vi "Argmin_min.vi"(6 "Type Y":enum16{"Array", "Sparse"}(ring), 7 "Type X":enum16{"Array", "Sparse"}(ring), 8 "error in":errorcluster caption="entrée d'erreur", 9 "Y":string[][](array[string]), 10 "X":string[][](array[string]), 11 "pairwise_distances_argmin_min":T2={"axis"=1, "metric "="euclidean", "metric_kwargs"={"metric"=[], "kwargs"=[]}, "Returns"="argmin"}) -> (0 "error out":errorcluster caption="sortie d'erreur", 3 "Data":T1)   [LabVIEW 2020]
uses:
  Argmin_min.lvclass
panel:
  out "Argmin_min.lvclass":refnum<class "Argmin_min.lvclass">
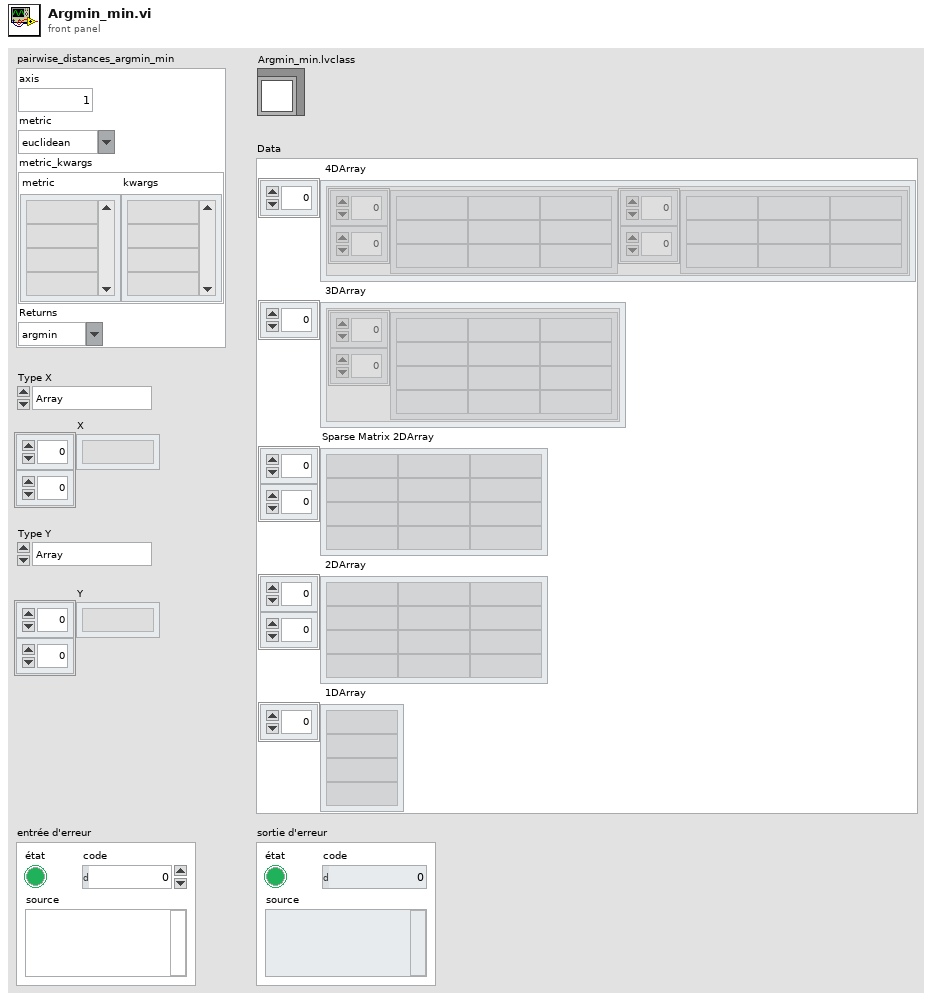
[diagram p1: front panel]
types:
  T1 = cluster{" 4DArray":cluster{"1":string[][], "2":string[][]}[], " 3DArray":cluster{"Tableau":string[][]}[], "Sparse Matrix 2DArray":string[][], " 2DArray":string[][], " 1DArray":string[]}
  T2 = cluster{"axis":i32, "metric ":string, "metric_kwargs":cluster{"metric":string[], "kwargs":string[]}, "Returns":string}
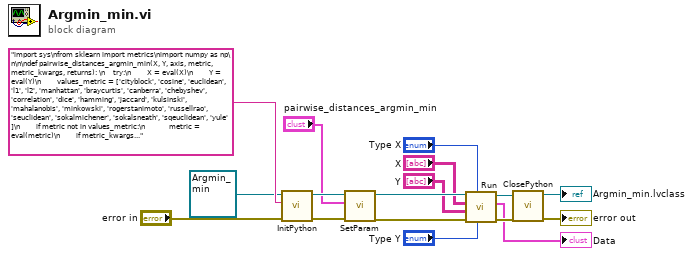
[diagram p0: block diagram]
diagram:
  n1 = call-dynamic "InitPython.vi"("error in (no error)"="error in", "Python Instruction"="import sys\nfrom sklearn import metrics\nimport numpy as np\n\n\ndef pairwise_distances_argmin_min(X, Y, axis, metric, metric_kwargs, returns): \n    try:\n        X = eval(X)\n        Y = eval(Y)\n        values_metric = ['cityblock', 'cosine', 'euclidean', 'l1', 'l2', 'manhattan', 'braycurtis', 'canberra', 'chebyshev', 'correlation', 'dice', 'hamming', 'jaccard', 'kulsinski', 'mahalanobis', 'minkowski', 'rogerstanimoto', 'russellrao', 'seuclidean', 'sokalmichener', 'sokalsneath', 'sqeuclidean', 'yule' ]\n        if metric not in values_metric:\n            metric = eval(metric)\n        if metric_kwargs == '':\n            metric_kwargs = None\n        else:\n            metric_kwargs= eval(metric_kwargs) \n        argmin, distances = metrics.pairwise_distances_argmin_min(X, Y, axis, metric, metric_kwargs)\n        if returns == 'argmin':\n            argmin = argmin.tolist()\n            return str(argmin)\n        else: \n            distances = distances.tolist()\n            return str(distances)\n    except:\n        erreur = sys.exc_info()\n        typerr = u\"%s\" % (erreur[0])\n        typerr = typerr[typerr.find(\"'\")+1:typerr.rfind(\"'\")]\n        msgerr = u\"%s\" % (erreur[1])\n        message = str('/!\\\\ {0} : {1}'. format(typerr,msgerr))\n        return message", "Scikit-learn en entrée"=refnum<class "Argmin_min.lvclass"> refnum ("Argmin_min.lvclass")) -> ("error out"=w14:errorcluster, "Scikit-learn en sortie"=w13:refnum<class "Argmin_min.lvclass">)  [unwired: 7 in]
  n2 = call-dynamic "SetParam.vi"("error in (no error)"=w14, "pairwise_distances_argmin_min"="pairwise_distances_argmin_min", "Argmin_min.lvclass"=w13) -> ("error out"=w10:errorcluster, "Argmin_min.lvclass"=w11:refnum<class "Argmin_min.lvclass">)  [unwired: 7 in]
  n3 = call-dynamic "Run.vi"("Type Y"="Type Y", "Type X"="Type X", "error in (no error)"=w10, "Y"="Y", "X"="X", "Argmin_min.lvclass"=w11) -> ("error out"=w8:errorcluster, "Data"=→"Data":T1, "Argmin_min.lvclass"=w9:refnum<class "Argmin_min.lvclass">)  [unwired: 3 in]
  n4 = call-dynamic "ClosePython.vi"("error in (no error)"=w8, "Scikit-learn en entrée"=w9) -> ("error out"=→"error out":errorcluster, "Scikit-learn en sortie"=→"Argmin_min.lvclass":refnum<class "Argmin_min.lvclass">)  [unwired: 8 in]
